vi "bats.parser.vi"(9 "time":u64, 10 "data.stream":T1={"data"=[0, 0, 0, 0, 0, 0, 0, 0], "data valid"=FALSE, "byte enables"=[FALSE, FALSE, FALSE, FALSE, FALSE, FALSE, FALSE, FALSE], "eof.good"=FALSE, "eof.bad"=FALSE, "frame.start"=0}, 11 "reset":bool) -> (2 "Ready.for.Udp.Input":bool)   [LabVIEW 2020]
uses:
  Market.Data.Common/fpga/my.network.data.stream.ctl
  bats.parser.state.data.ctl
  bats.parser.state.command.ctl
  Market.Data.Common/fpga/debug.data.cmd.ctl
  Market.Data.Common/fpga/debug.data.cmd.type.ctl
  <vilib>/rvi/Emulation/niFpgaEmulationIsFPGAContextNoSignature.vi
  <vilib>/rvi/Emulation/niFpgaSctlEmulationGetInTimedLoop.vi
  <vilib>/rvi/errors/niFpgaSetErrorForExecOnDevCompSimple.vi
  <vilib>/rvi/eio/common/nirviEmuReportErrorAndStop.vi
  <vilib>/rvi/DataTransferAndStorage/Container/Common/niFpgaContainerGetUniqueNameForEmu.vi
  <vilib>/rvi/FIFO/Fifo_Resource/nirvififoEmulationSetSize.vi
  <vilib>/rvi/FIFO/Fifo_Resource/nirviFifoEmulationQueueMgr.vi
  <instcachedir>/0/nirviFifoEmulationQueueMgr_E5CAEC123FF24DC58D834DCA3CDAA9B5.lvgen/nirviFifoEmulationQueueMgr_E5CAEC123FF24DC58D834DCA3CDAA9B5_020.vi
  <vilib>/rvi/FIFO/Fifo_Resource/nirvififoEmulationDetermineInputValidOut.vi
  <vilib>/rvi/FIFO/Fifo_Resource/nirvififoEmulationCreateLock.vi
  <vilib>/rvi/Emulation/niFpgaProcessEmulError.vi
  <vilib>/rvi/FIFO/Fifo_Resource/nirvififoEmulationObtainLock.vi
  <vilib>/rvi/FIFO/Fifo_Resource/nirvififoEmulationReleaseLock.vi
  <vilib>/rvi/occurrence/nirviWaitOnOccurrenceBase.vi
  <vilib>/rvi/errors/nirviReportUnexpectedCaseInternalError.vi
  <vilib>/rvi/errors/nirviReportUnexpectedCaseInternalError (U32).vi
  <instcachedir>/0/nirviFifoEmulationQueueMgr_E5CAEC123FF24DC58D834DCA3CDAA9B5.lvgen/nirviFifoEmulationQueueMgr_E5CAEC123FF24DC58D834DCA3CDAA9B5_017.vi
  <vilib>/rvi/DataTransferAndStorage/Container/XNode/niFpgaContainer.xnode
  <vilib>/rvi/FIFO/Fifo_Resource/nirvififoEmulationWrite.vi
  Market.Data.Common/fpga/fpganow.common.fpga.lvlib
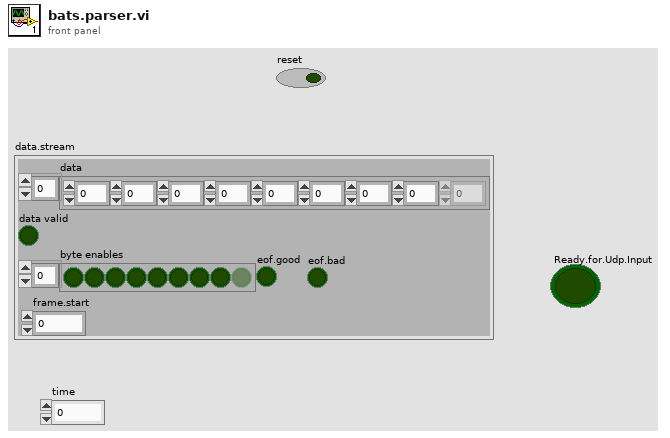
[diagram p1: front panel]
types:
  T1 = typedef "my.network.data.stream.ctl" = cluster{"data":u8[], "data valid":bool, "byte enables":bool[], "eof.good":bool, "eof.bad":bool, "frame.start":u64}
  T2 = typedef "bats.parser.state.command.ctl" = enum16{"Reset", "Noop", "Read.Sequenced.Unit.Header", "Read.Msg"}
  T3 = typedef "bats.parser.state.data.ctl" = cluster{"BATS.Parser.States":T2, "Saved.BATS.Parser.State":T2, "Hdr Length (U16)":u16, "MessageLength (U8)":u8, "MessageType (U8)":u8, "Time (U32)":u32, "Total Counter (U16)":u16, "Message Counter (U8)":u8, "i":u16, "Number.of.Tickers":u16, "n":u16, "msg.counter":u8, "msg.length":u8, "buffer.start":u8, "buffer.length":u8, "buffer":u64[], "Next.Seq.No":u32, "debug":T4}
  T4 = typedef "fpganow.common.fpga.lvlib/debug.data.cmd.ctl" = cluster{"write":bool, "data":T5}
  T5 = typedef "fpganow.common.fpga.lvlib/debug.data.cmd.type.ctl" = u64[]
  T6 = typedef "fpganow.common.fpga.lvlib/orderbook.command.ctl" = cluster{"type":T7, "side":u8, "orderId ":u64, "quantity":u32, "symbol":u64, "price":u64, "executed.qty":u32, "canceled.qty":u32, "remaining.qty":u32, "seconds":u64, "nanoseconds":u64, "Add":bool, "Edit":bool, "Remove":bool, "seq no":u32, "recv.time":u64, "parse.time":u64}
  T7 = typedef "fpganow.common.fpga.lvlib/orderbook.command.type.ctl" = enum8{"Time", "AddOrder", "OrderExecuted", "OrderExecutedAtPrice", "ReduceSize", "ModifyOrder", "DeleteOrder", "Get.Everything", "Get.All.Orders", "Get.Top"}
  T8 = cluster{"type":enum8{"Time", "AddOrder", "OrderExecuted", "OrderExecutedAtPrice", "ReduceSize", "ModifyOrder", "DeleteOrder", "Get.Everything", "Get.All.Orders", "Get.Top"}, "side":u8, "orderId ":u64, "quantity":u32, "symbol":u64, "price":u64, "executed.qty":u32, "canceled.qty":u32, "remaining.qty":u32, "seconds":u64, "nanoseconds":u64, "Add":bool, "Edit":bool, "Remove":bool, "seq no":u32, "recv.time":u64, "parse.time":u64}
  T9 = cluster{"type":enum8{"Time", "AddOrder", "OrderExecuted", "OrderExecutedAtPrice", "ReduceSize", "ModifyOrder", "DeleteOrder", "Get.Everything", "Get.All.Orders", "Get.Top", "Trade", "Unsupported"}, "side":u8, "orderId ":u64, "quantity":u32, "symbol":u64, "price":u64, "executed.qty":u32, "canceled.qty":u32, "remaining.qty":u32, "seconds":u64, "nanoseconds":u64, "Add":bool, "Edit":bool, "Remove":bool, "seq no":u32, "recv.time":u64, "parse.time":u64}
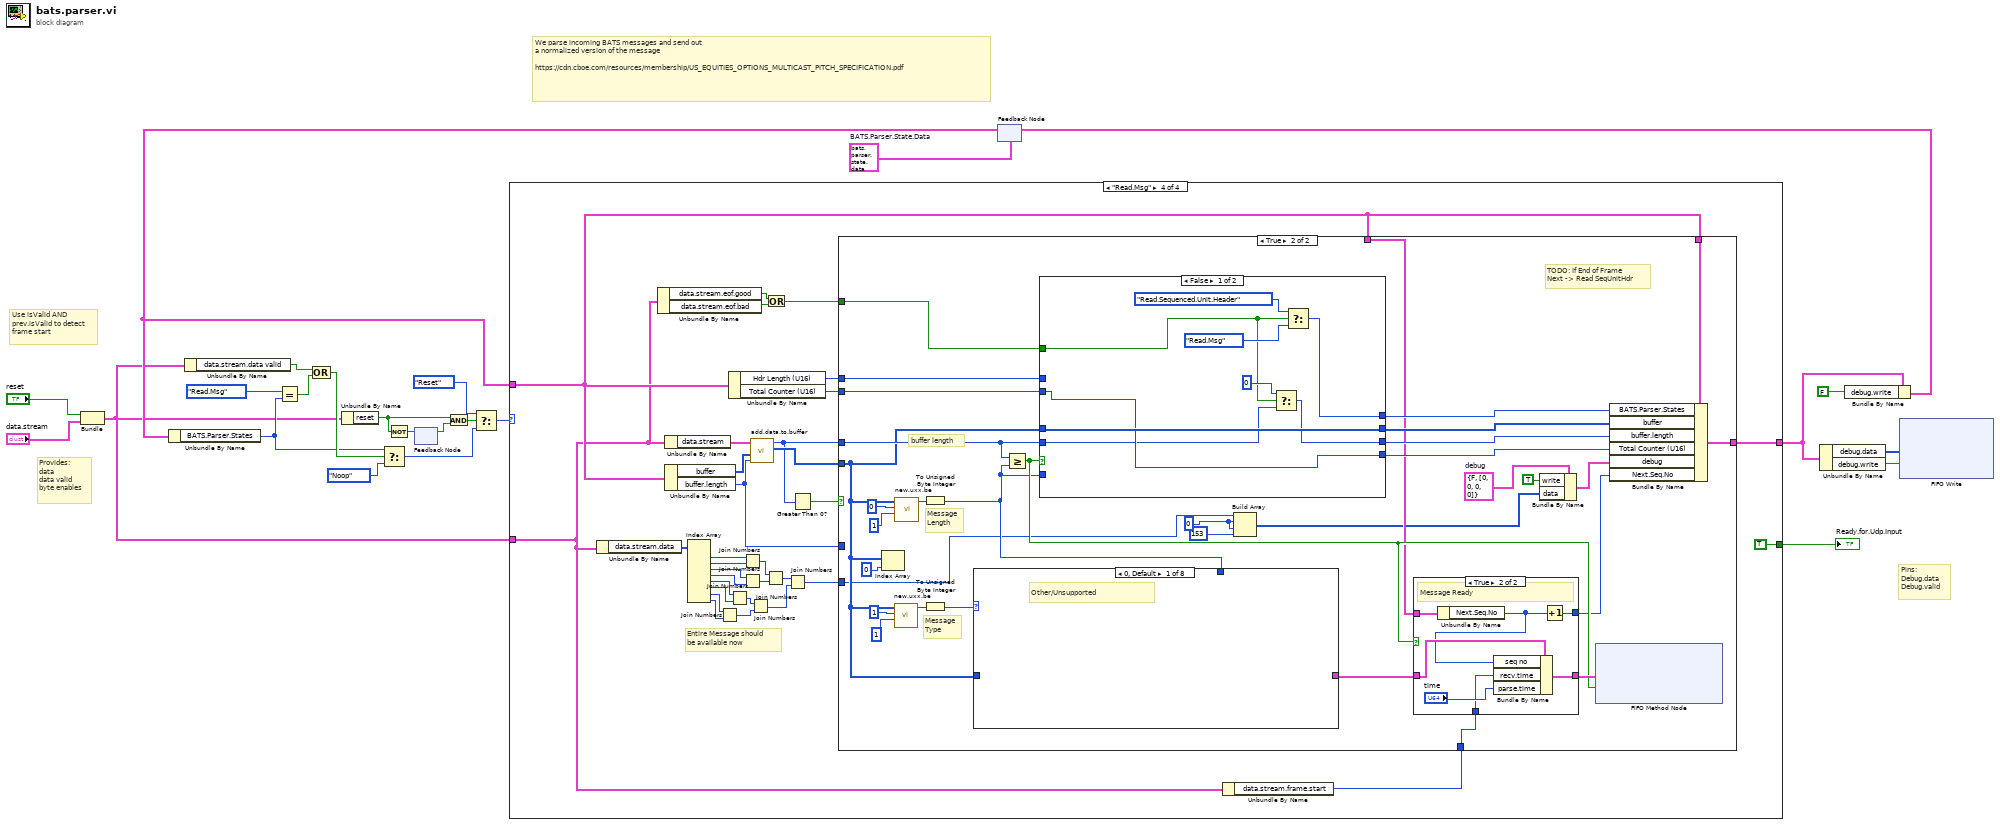
[diagram p0: block diagram]
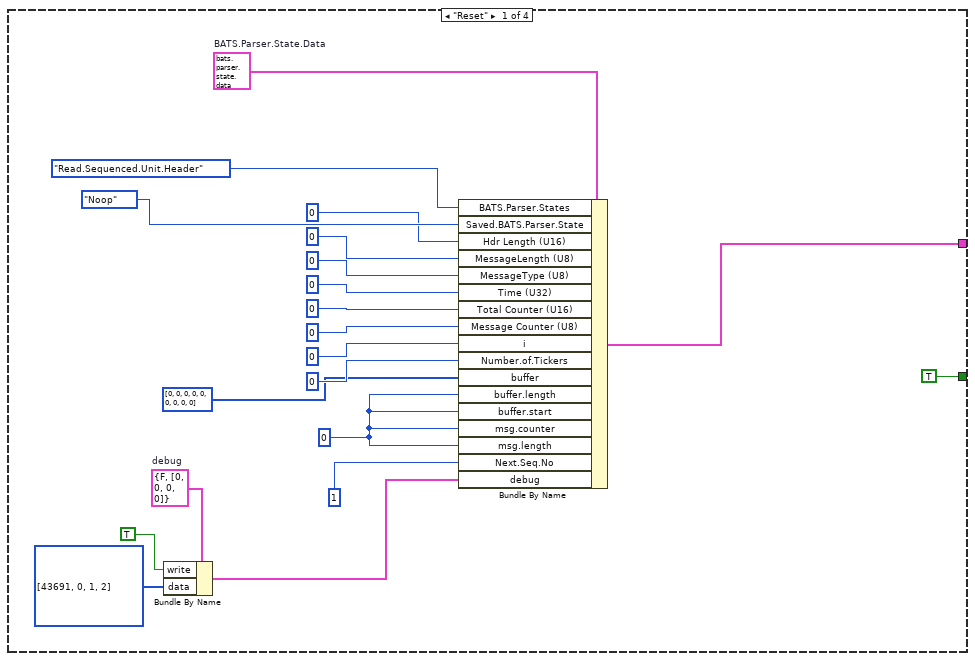
[diagram p2: hidden frame]
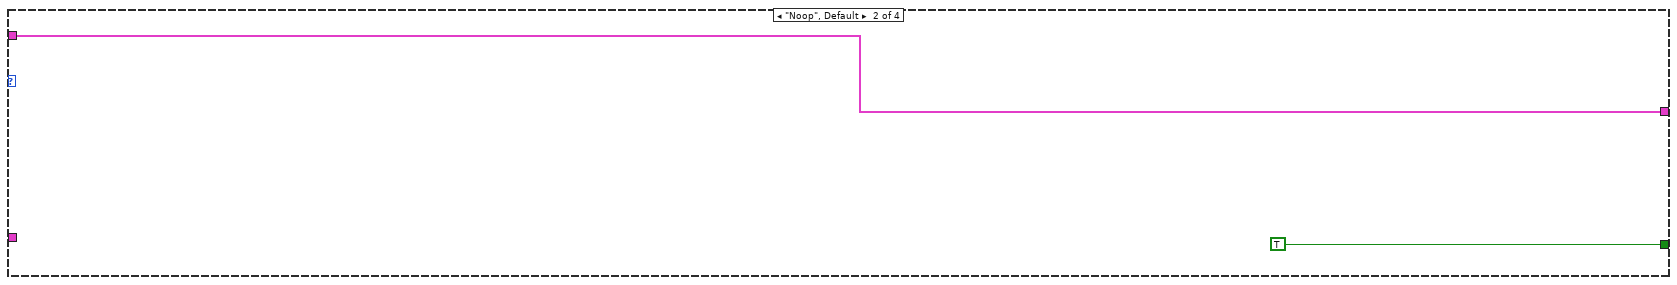
[diagram p3: hidden frame]
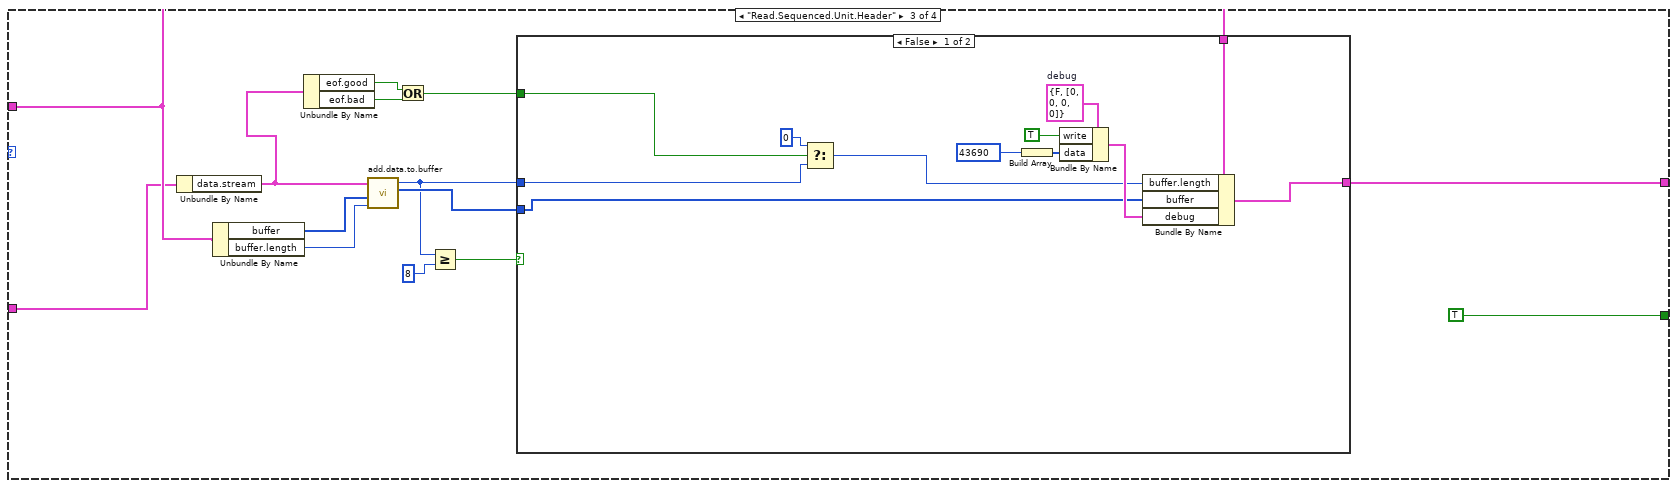
[diagram p4: hidden frame]
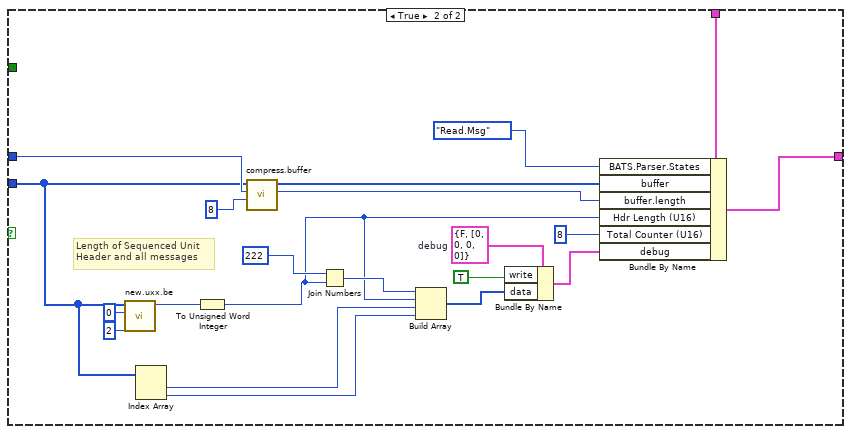
[diagram p5: hidden frame]
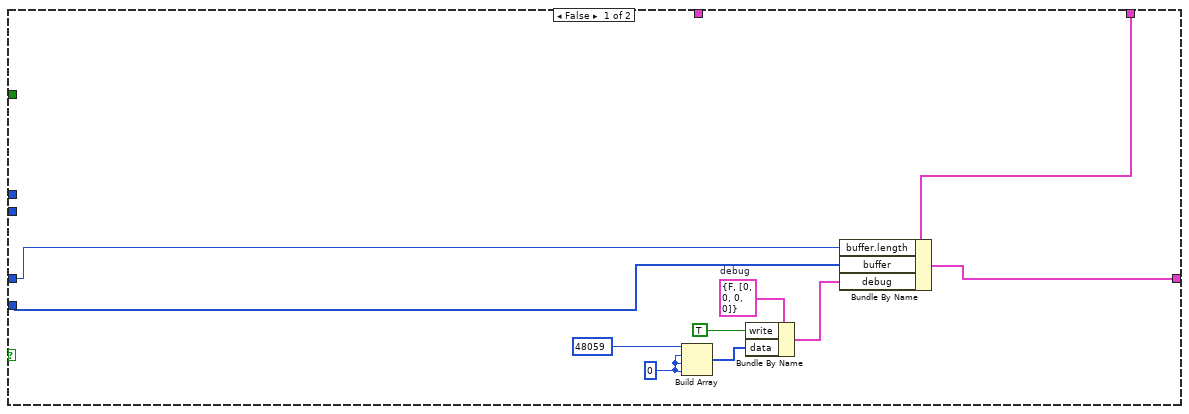
[diagram p6: hidden frame]
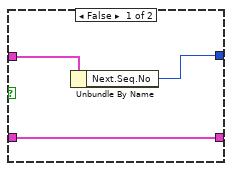
[diagram p7: hidden frame]
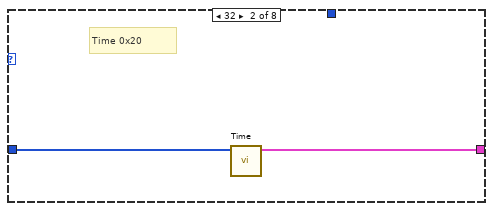
[diagram p8: hidden frame]
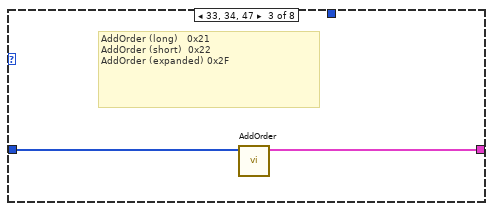
[diagram p9: hidden frame]
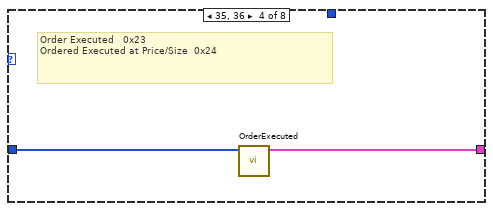
[diagram p10: hidden frame]
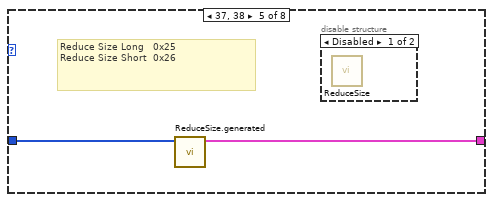
[diagram p11: hidden frame]
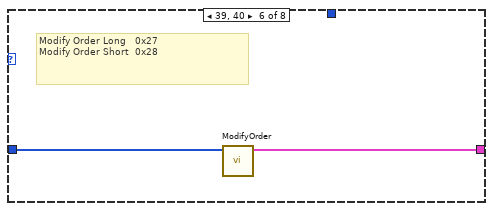
[diagram p13: hidden frame]
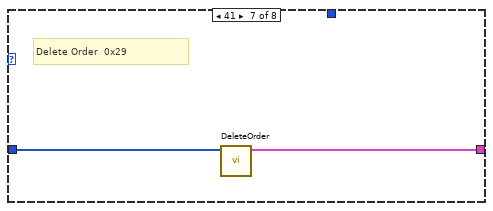
[diagram p14: hidden frame]
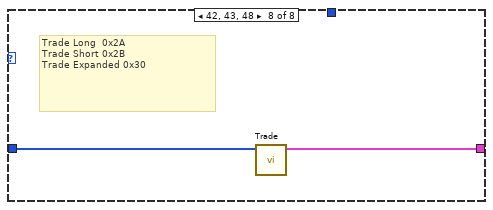
[diagram p15: hidden frame]
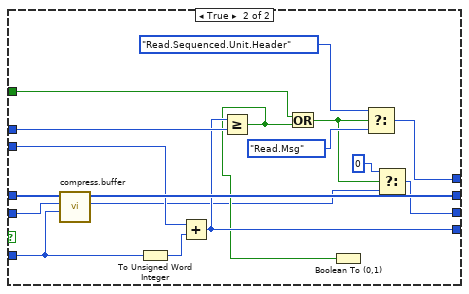
[diagram p16: hidden frame]
diagram:
  w24 = T3 {"BATS.Parser.States"=enum."Read.Sequenced.Unit.Header", "Saved.BATS.Parser.State"=enum."Reset", "Hdr Length (U16)"=0, "MessageLength (U8)"=0, "MessageType (U8)"=0, "Time (U32)"=0, "Total Counter (U16)"=0, "Message Counter (U8)"=0, "i"=0, "Number.of.Tickers"=0, "n"=0, "msg.counter"=0, "msg.length"=0, "buffer.start"=0, "buffer.length"=0, "buffer"=[0, 0, 0, 0, 0, 0, 0, 0, 0], "Next.Seq.No"=0, "debug"={"write"=FALSE, "data"=[0, 0, 0, 0]}}  # BATS.Parser.State.Data
  # "Use isValid AND\nprev.isValid to detect\nframe start"
  # "Provides:\ndata\ndata valid\nbyte enables"
  # "Pins:\nDebug.data\nDebug.valid"
  # "We parse incoming BATS messages and send out\na normalized version of the message\n\nhttps://cdn.cboe.com/resources/membership/US_EQUITIES_OPTIONS_MULTICAST_PITCH_SPECIFICATION.pdf"
  n1 = Bundle("reset"="reset", "data.stream"="data.stream") -> (w1:cluster{"reset":bool, "data.stream":T1})  [unwired: 1 in]
  n2 = Unbundle By Name(w1) -> ("data.stream.data valid"=w11:bool)
  n3 = Unbundle By Name(w1) -> ("reset"=w14:bool)
  n4 = Not(x=w14) -> (.not. x?=w16:bool)
  n5 = feedback-in #1(w16) -> ()
  n6 = feedback #1() -> (w17:bool)  [unwired: 1 in]
  n7 = And(x=w14, y=w17) -> (x .and. y?=w18:bool)
  n8 = feedback #2(w24) -> (w4:T3)
  n9 = Unbundle By Name(w4) -> ("BATS.Parser.States"=w8:T2)
  n10 = Equal?(x=bats.parser.state.command."Read.Msg" ("BATS.Parser.States"), y=w8) -> (x = y?=w19:bool)
  n11 = Compound Arithmetic op=OR(w11, w19) -> (w10:bool)
  n12 = Select(t=w8, s=w10, f=bats.parser.state.command."Noop" ("BATS.Parser.States")) -> (s? t:f=w9:T2)
  n13 = Select(t=bats.parser.state.command."Reset" ("BATS.Parser.States"), s=w18, f=w9) -> (s? t:f=w21:T2)
  n14 = case shown="\"Read.Msg\"" w21 {
    tunnel: w4 -> [_ w46 w56 w117]
    tunnel: [w43 w46 w58 w125] -> w5
    tunnel: [TRUE ("Ready for Input") TRUE ("Ready for Input") TRUE ("Ready for Input") TRUE ("Ready for Input")] -> w15
    tunnel: w1 -> [_ _ w51 w97]
    frame "Reset" {
      w26 = T4 {"write"=FALSE, "data"=[0, 0, 0, 0]}  # debug
      w28 = u8 0 ("buffer.length")
      w44 = T3 {"BATS.Parser.States"=enum."Read.Sequenced.Unit.Header", "Saved.BATS.Parser.State"=enum."Reset", "Hdr Length (U16)"=0, "MessageLength (U8)"=0, "MessageType (U8)"=0, "Time (U32)"=0, "Total Counter (U16)"=0, "Message Counter (U8)"=0, "i"=0, "Number.of.Tickers"=0, "n"=0, "msg.counter"=0, "msg.length"=0, "buffer.start"=0, "buffer.length"=0, "buffer"=[0, 0, 0, 0, 0, 0, 0, 0, 0], "Next.Seq.No"=0, "debug"={"write"=FALSE, "data"=[0, 0, 0, 0]}}  # BATS.Parser.State.Data
      n15 = Bundle By Name(cluster=w26, "write"=TRUE ("Write.to.Debug"), "data"=u64[] [43691, 0, 1, 2] ("appended array")) -> (w29:T4)
      n16 = Bundle By Name(cluster=w44, "BATS.Parser.States"=bats.parser.state.command."Read.Sequenced.Unit.Header", "Saved.BATS.Parser.State"=bats.parser.state.command."Noop" ("BATS.Parser.States"), "Hdr Length (U16)"=u16 0, "MessageLength (U8)"=u8 0, "MessageType (U8)"=u8 0, "Time (U32)"=u32 0, "Total Counter (U16)"=u16 0, "Message Counter (U8)"=u8 0, "i"=u16 0, "Number.of.Tickers"=u16 0, "buffer"=u64[] [0, 0, 0, 0, 0, 0, 0, 0, 0], "buffer.length"=w28, "buffer.start"=w28, "msg.counter"=w28, "msg.length"=w28, "Next.Seq.No"=u32 1, "debug"=w29) -> (w43:T3)
    }
    frame "Noop", Default {
    }
    frame "Read.Sequenced.Unit.Header" {
      n17 = Unbundle By Name(w51) -> ("data.stream"=w50:T1)
      n18 = Unbundle By Name(w56) -> ("buffer"=w60:u64[], "buffer.length"=w59:u8)
      n19 = Unbundle By Name(w50) -> ("eof.good"=w48:bool, "eof.bad"=w49:bool)
      n20 = call "add.data.to.buffer.vi"("buffer.length"=w59, "buffer"=w60, "data.stream"=w50) -> ("buffer.out"=w57:u64[], "buffer.length.out"=w54:u8)  [unwired: 7 in]
      n21 = Or(x=w48, y=w49) -> (x .or. y?=w47:bool)
      n22 = Greater Or Equal?(x=w54, y=u8 8) -> (x >= y?=w55:bool)
      n23 = case shown="False" w55 {
        tunnel: [w70 w93] -> w58
        tunnel: w57 -> [w68 w75]
        tunnel: w54 -> [w62 w82]
        tunnel: w56 -> [w69 w91]
        tunnel: w47 -> [w64 _]
        frame False {
          w66 = T4 {"write"=FALSE, "data"=[0, 0, 0, 0]}  # debug
          n24 = Select(t=u8 0, s=w64, f=w62) -> (s? t:f=w61:u8)
          n25 = Build Array(u64 43690 ("Data")) -> (w65:u64[])
          n26 = Bundle By Name(cluster=w66, "write"=TRUE ("Write.to.Debug"), "data"=w65) -> (w72:T4)
          n27 = Bundle By Name(cluster=w69, "buffer.length"=w61, "buffer"=w68, "debug"=w72) -> (w70:T3)
        }
        frame True {
          w78 = T4 {"write"=FALSE, "data"=[0, 0, 0, 0]}  # debug
          # "Length of Sequenced Unit\nHeader and all messages"
          n28 = call "new.uxx.be.vi"("buffer (U64)"=w75, "Start.Idx"=u8 0, "Length"=u8 2) -> ("Out.Value U64"=w86:u64)  [unwired: 7 in]
          n29 = Index Array(array=w75) -> (element #1=w74:u64, element #2=w73:u64)  [unwired: 2 in]
          n30 = To Unsigned Word Integer(number=w86) -> (unsigned 16bit integer=w76:u16)
          n31 = call "compress.buffer.vi"("start.idx"=u8 8, "buffer.length"=w82, "buffer"=w75) -> ("buffer.length.out"=w81:u8, "buffer.out"=w87:u64[])  [unwired: 7 in]
          n32 = Join Numbers(hi=u32 222 ("Data"), lo=w76) -> ((hi.lo)=w79:u64)
          n33 = Build Array(w79, w76, w74, w73) -> (w77:u64[])
          n34 = Bundle By Name(cluster=w78, "write"=TRUE ("Write.to.Debug"), "data"=w77) -> (w84:T4)
          n35 = Bundle By Name(cluster=w91, "BATS.Parser.States"=bats.parser.state.command."Read.Msg", "buffer"=w87, "buffer.length"=w81, "Hdr Length (U16)"=w76, "Total Counter (U16)"=u16 8, "debug"=w84) -> (w93:T3)
        }
      }
    }
    frame "Read.Msg" {
      # "Entire Message should \nbe available now"
      n36 = Unbundle By Name(w97) -> ("data.stream.data"=w100:u8[])
      n37 = Unbundle By Name(w97) -> ("data.stream.eof.good"=w96:bool, "data.stream.eof.bad"=w95:bool)
      n38 = Unbundle By Name(w97) -> ("data.stream"=w99:T1)
      n39 = Unbundle By Name(w117) -> ("buffer"=w116:u64[], "buffer.length"=w119:u8)
      n40 = Index Array(array=w100) -> (element #1=w115:u8, element #2=w114:u8, element #3=w113:u8, element #4=w112:u8, element #5=w111:u8, element #6=w110:u8, element #7=w109:u8, element #8=w108:u8)  [unwired: 8 in]
      n41 = Join Numbers(hi=w109, lo=w108) -> ((hi.lo)=w107:u16)
      n42 = Unbundle By Name(w117) -> ("Hdr Length (U16)"=w121:u16, "Total Counter (U16)"=w120:u16)
      n43 = Join Numbers(hi=w111, lo=w110) -> ((hi.lo)=w106:u16)
      n44 = Join Numbers(hi=w115, lo=w114) -> ((hi.lo)=w104:u16)
      n45 = Join Numbers(hi=w113, lo=w112) -> ((hi.lo)=w105:u16)
      n46 = Join Numbers(hi=w106, lo=w107) -> ((hi.lo)=w102:u32)
      n47 = call "add.data.to.buffer.vi"("buffer.length"=w119, "buffer"=w116, "data.stream"=w99) -> ("buffer.out"=w124:u64[], "buffer.length.out"=w123:u8)  [unwired: 7 in]
      n48 = Or(x=w96, y=w95) -> (x .or. y?=w94:bool)
      n49 = Join Numbers(hi=w104, lo=w105) -> ((hi.lo)=w103:u32)
      n50 = Join Numbers(hi=w103, lo=w102) -> ((hi.lo)=w101:u64)
      n51 = Greater Than 0?(x=w123) -> (x > 0?=w122:bool)
      n52 = Unbundle By Name(w97) -> ("data.stream.frame.start"=w98:u64)
      n53 = case shown="True" w122 {
        tunnel: [w134 w168] -> w125
        tunnel: w124 -> [w133 w143]
        tunnel: w123 -> [w130 w154]
        tunnel: w117 -> [w135 w167]
        tunnel: w121 -> [_ w157]
        tunnel: w120 -> [_ w156]
        tunnel: w119 -> [_ _]
        tunnel: w117 -> [_ w145]
        tunnel: w101 -> [_ w141]
        tunnel: w98 -> [_ w138]
        tunnel: w94 -> [_ w137]
        frame False {
          w126 = u64 0 ("element")
          w128 = T4 {"write"=FALSE, "data"=[0, 0, 0, 0]}  # debug
          n54 = Build Array(u64 48059 ("Data"), w126, w126, w126) -> (w127:u64[])
          n55 = Bundle By Name(cluster=w128, "write"=TRUE ("Write.to.Debug"), "data"=w127) -> (w132:T4)
          n56 = Bundle By Name(cluster=w135, "buffer.length"=w130, "buffer"=w133, "debug"=w132) -> (w134:T3)
        }
        frame True {
          w139 = u64 0 ("element")
          w136 = T4 {"write"=FALSE, "data"=[0, 0, 0, 0]}  # debug
          # "TODO: If End of Frame\nNext -> Read SeqUnitHdr"
          # "buffer length"
          # "Message\nType"
          # "Message\nLength"
          n57 = Index Array(array=w143, index=0) -> ()  [unwired: 1 out]
          n58 = call "new.uxx.be.vi"("buffer (U64)"=w143, "Start.Idx"=u8 1, "Length"=u8 1) -> ("Out.Value U64"=w162:u64)  [unwired: 7 in]
          n59 = call "new.uxx.be.vi"("buffer (U64)"=w143, "Start.Idx"=u8 0, "Length"=u8 1) -> ("Out.Value U64"=w164:u64)  [unwired: 7 in]
          n60 = To Unsigned Byte Integer(number=w164) -> (unsigned 8bit integer=w144:u8)
          n61 = To Unsigned Byte Integer(number=w162) -> (unsigned 8bit integer=w151:u8)
          n62 = case shown="0, Default" w151 {
            tunnel: [_ w179 w182 w184 w185 w188 w190 w191] -> w149
            tunnel: w143 -> [_ w180 w181 w183 w186 w187 w189 w192]
            tunnel: w144 -> [_ _ _ _ _ _ _ _]
            frame 0, Default {
              # "Other/Unsupported"
            }
            frame 32 {
              # "Time 0x20"
              n63 = call "Time.vi"("buffer.in"=w180) -> ("OrderBook.Command"=w179:T6)  [unwired: 10 in]
            }
            frame 33, 34, 47 {
              # "AddOrder (long)   0x21\nAddOrder (short)  0x22\nAddOrder (expanded) 0x2F"
              n64 = call "AddOrder.vi"("buffer.in"=w181) -> ("OrderBook.Command"=w182:T6)  [unwired: 10 in]
            }
            frame 35, 36 {
              # "Order Executed   0x23\nOrdered Executed at Price/Size  0x24"
              n65 = call "OrderExecuted.vi"("buffer.in"=w183) -> ("OrderBook.Command"=w184:T6)  [unwired: 10 in]
            }
            frame 37, 38 {
              # "Reduce Size Long   0x25\nReduce Size Short  0x26"
              n66 = call "ReduceSize.generated.vi"("buffer.in"=w186) -> ("OrderBook.Command"=w185:T8)  [unwired: 10 in]
              n67 = disable-structure shown="Disabled" {
                frame Disabled {
                  n68 = call "ReduceSize.vi"() -> ()  [unwired: 11 in, 1 out]
                }
                frame Enabled {
                }
              }
            }
            frame 39, 40 {
              # "Modify Order Long   0x27\nModify Order Short  0x28"
              n69 = call "ModifyOrder.vi"("buffer.in"=w187) -> ("OrderBook.Command"=w188:T8)  [unwired: 10 in]
            }
            frame 41 {
              # "Delete Order  0x29"
              n70 = call "DeleteOrder.vi"("buffer.in"=w189) -> ("OrderBook.Command"=w190:T8)  [unwired: 10 in]
            }
            frame 42, 43, 48 {
              # "Trade Long  0x2A\nTrade Short 0x2B\nTrade Expanded 0x30"
              n71 = call "Trade.vi"("buffer.in"=w192) -> ("OrderBook.Command"=w191:T9)  [unwired: 10 in]
            }
          }
          n72 = Greater Or Equal?(x=w154, y=w144) -> (x >= y?=w147:bool)
          n73 = case shown="False" w147 {
            tunnel: [w193 w205] -> w160
            tunnel: [w201 w218] -> w161
            tunnel: w154 -> [w196 w216]
            tunnel: w143 -> [w201 w217]
            tunnel: w144 -> [_ w215]
            tunnel: [w197 w210] -> w159
            tunnel: [w200 w208] -> w158
            tunnel: w157 -> [_ w212]
            tunnel: w156 -> [w200 w213]
            tunnel: w137 -> [w194 w206]
            frame False {
              n74 = Select(t=u8 0, s=w194, f=w196) -> (s? t:f=w193:u8)
              n75 = Select(t=bats.parser.state.command."Read.Sequenced.Unit.Header", s=w194, f=bats.parser.state.command."Read.Msg" ("BATS.Parser.States")) -> (s? t:f=w197:T2)
            }
            frame True {
              n76 = call "compress.buffer.vi"("start.idx"=w215, "buffer.length"=w216, "buffer"=w217) -> ("buffer.length.out"=w204:u8, "buffer.out"=w218:u64[])  [unwired: 7 in]
              n77 = To Unsigned Word Integer(number=w215) -> (unsigned 16bit integer=w214:u16)
              n78 = Add(x=w213, y=w214) -> (x+y=w208:u16)
              n79 = Greater Or Equal?(x=w208, y=w212) -> (x >= y?=w207:bool)
              n80 = Or(x=w206, y=w207) -> (x .or. y?=w203:bool)
              n81 = Boolean To (0,1)(Boolean=w207) -> ()  [unwired: 1 out]
              n82 = Select(t=bats.parser.state.command."Read.Sequenced.Unit.Header", s=w203, f=bats.parser.state.command."Read.Msg" ("BATS.Parser.States")) -> (s? t:f=w210:T2)
              n83 = Select(t=u8 0, s=w203, f=w204) -> (s? t:f=w205:u8)
            }
          }
          n84 = Build Array(w141, w139, w139, u64 153 ("element")) -> (w142:u64[])
          n85 = case shown="True" w147 {
            tunnel: w149 -> [w171 w178]
            tunnel: [w171 w177] -> w148
            tunnel: w145 -> [w169 w176]
            tunnel: [w170 w174] -> w146
            tunnel: w138 -> [_ w172]
            frame False {
              n86 = Unbundle By Name(w169) -> ("Next.Seq.No"=w170:u32)
            }
            frame True {
              # "Message Ready"
              n87 = Unbundle By Name(w176) -> ("Next.Seq.No"=w175:u32)
              n88 = Bundle By Name(cluster=w178, "seq no"=w175, "recv.time"=w172, "parse.time"="time") -> (w177:T9)
              n89 = Increment(x=w175) -> (x+1=w174:u32)
            }
          }
          n90 = Bundle By Name(cluster=w136, "write"=TRUE ("Write.to.Debug"), "data"=w142) -> (w155:T4)
          n91 = xnode ("FIFO Method Node")("Element"=w148, "Input Valid"=w147) -> ()  [unwired: 1 in, 2 out]
          n92 = Bundle By Name(cluster=w167, "BATS.Parser.States"=w159, "buffer"=w161, "buffer.length"=w160, "Total Counter (U16)"=w158, "debug"=w155, "Next.Seq.No"=w146) -> (w168:T3)
        }
      }
    }
  }
  "Ready.for.Udp.Input" <- w15
  n93 = Unbundle By Name(w5) -> ("debug.data"=w3:T5, "debug.write"=w6:bool)
  n94 = Bundle By Name(cluster=w5, "debug.write"=FALSE ("Debug.Write.to.Debug")) -> (w13:T3)
  n95 = feedback-in #2(w13) -> ()
  n96 = xnode ("FIFO Write")("Element"=w3, "Input Valid"=w6) -> ()  [unwired: 1 in, 2 out]
